vi "APDM Initialize Hardware.vi"(3 "error in (no error)":errorcluster, 4 "Gyro Sim Time Data":path=path "C:/Users/jfalesi/Desktop/CP FES Walking Code/Original/Ahad Vi/CP Code/Offline data/TD_7_time.txt", 5 "APDM Context in":T1) -> (0 "error out":errorcluster, 2 "APDM Context out":T1)   [LabVIEW 2019]
uses:
  Controls/APDM Context Cluster.ctl
  <vilib>/Utility/file.llb/Read Delimited Spreadsheet (DBL).vi
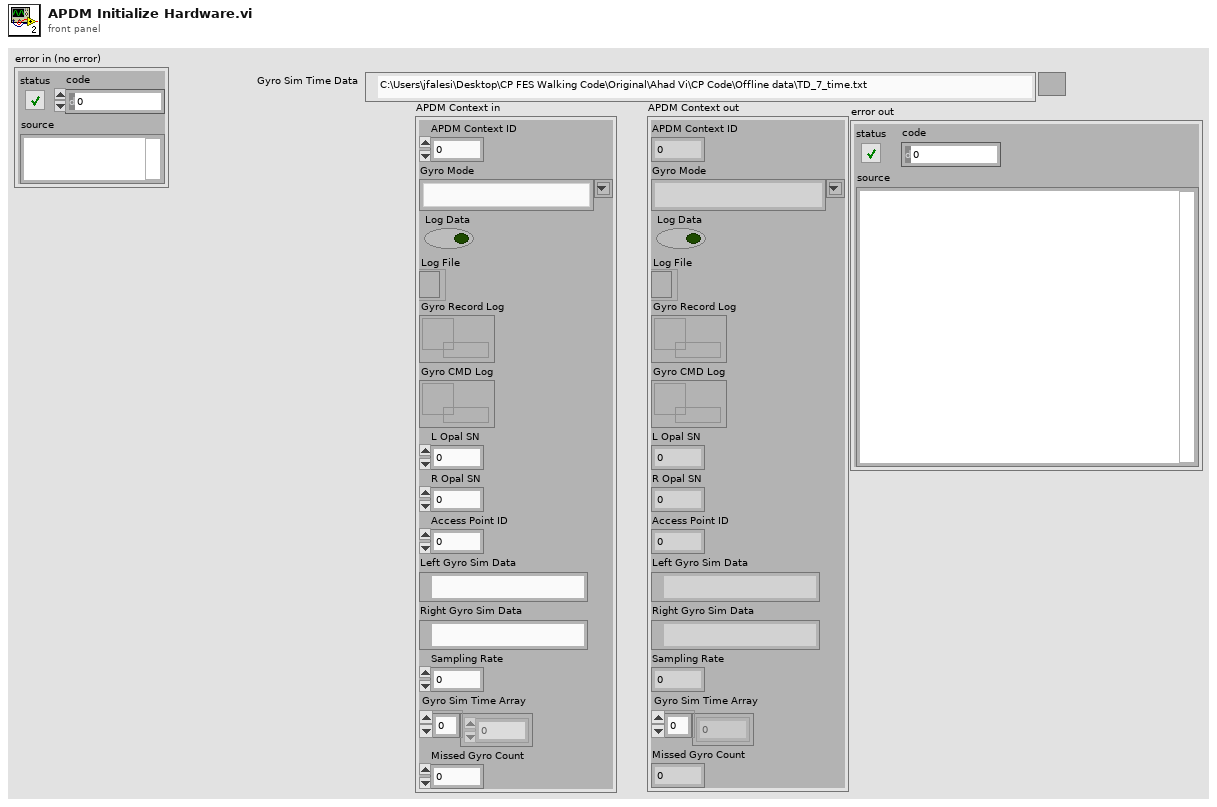
[diagram p1: front panel]
types:
  T1 = typedef "APDM Context Cluster.ctl" = cluster{"APDM Context ID":u32, "Gyro Mode":string, "Log Data":bool, "Log File":refnum<file>, "Gyro Record Log":refnum<queue>, "Gyro CMD Log":refnum<queue>, "L Opal SN":u32, "R Opal SN":u32, "Access Point ID":u32, "Left Gyro Sim Data":path, "Right Gyro Sim Data":path, "Sampling Rate":dbl, "Gyro Sim Time Array":dbl[], "Missed Gyro Count":dbl}
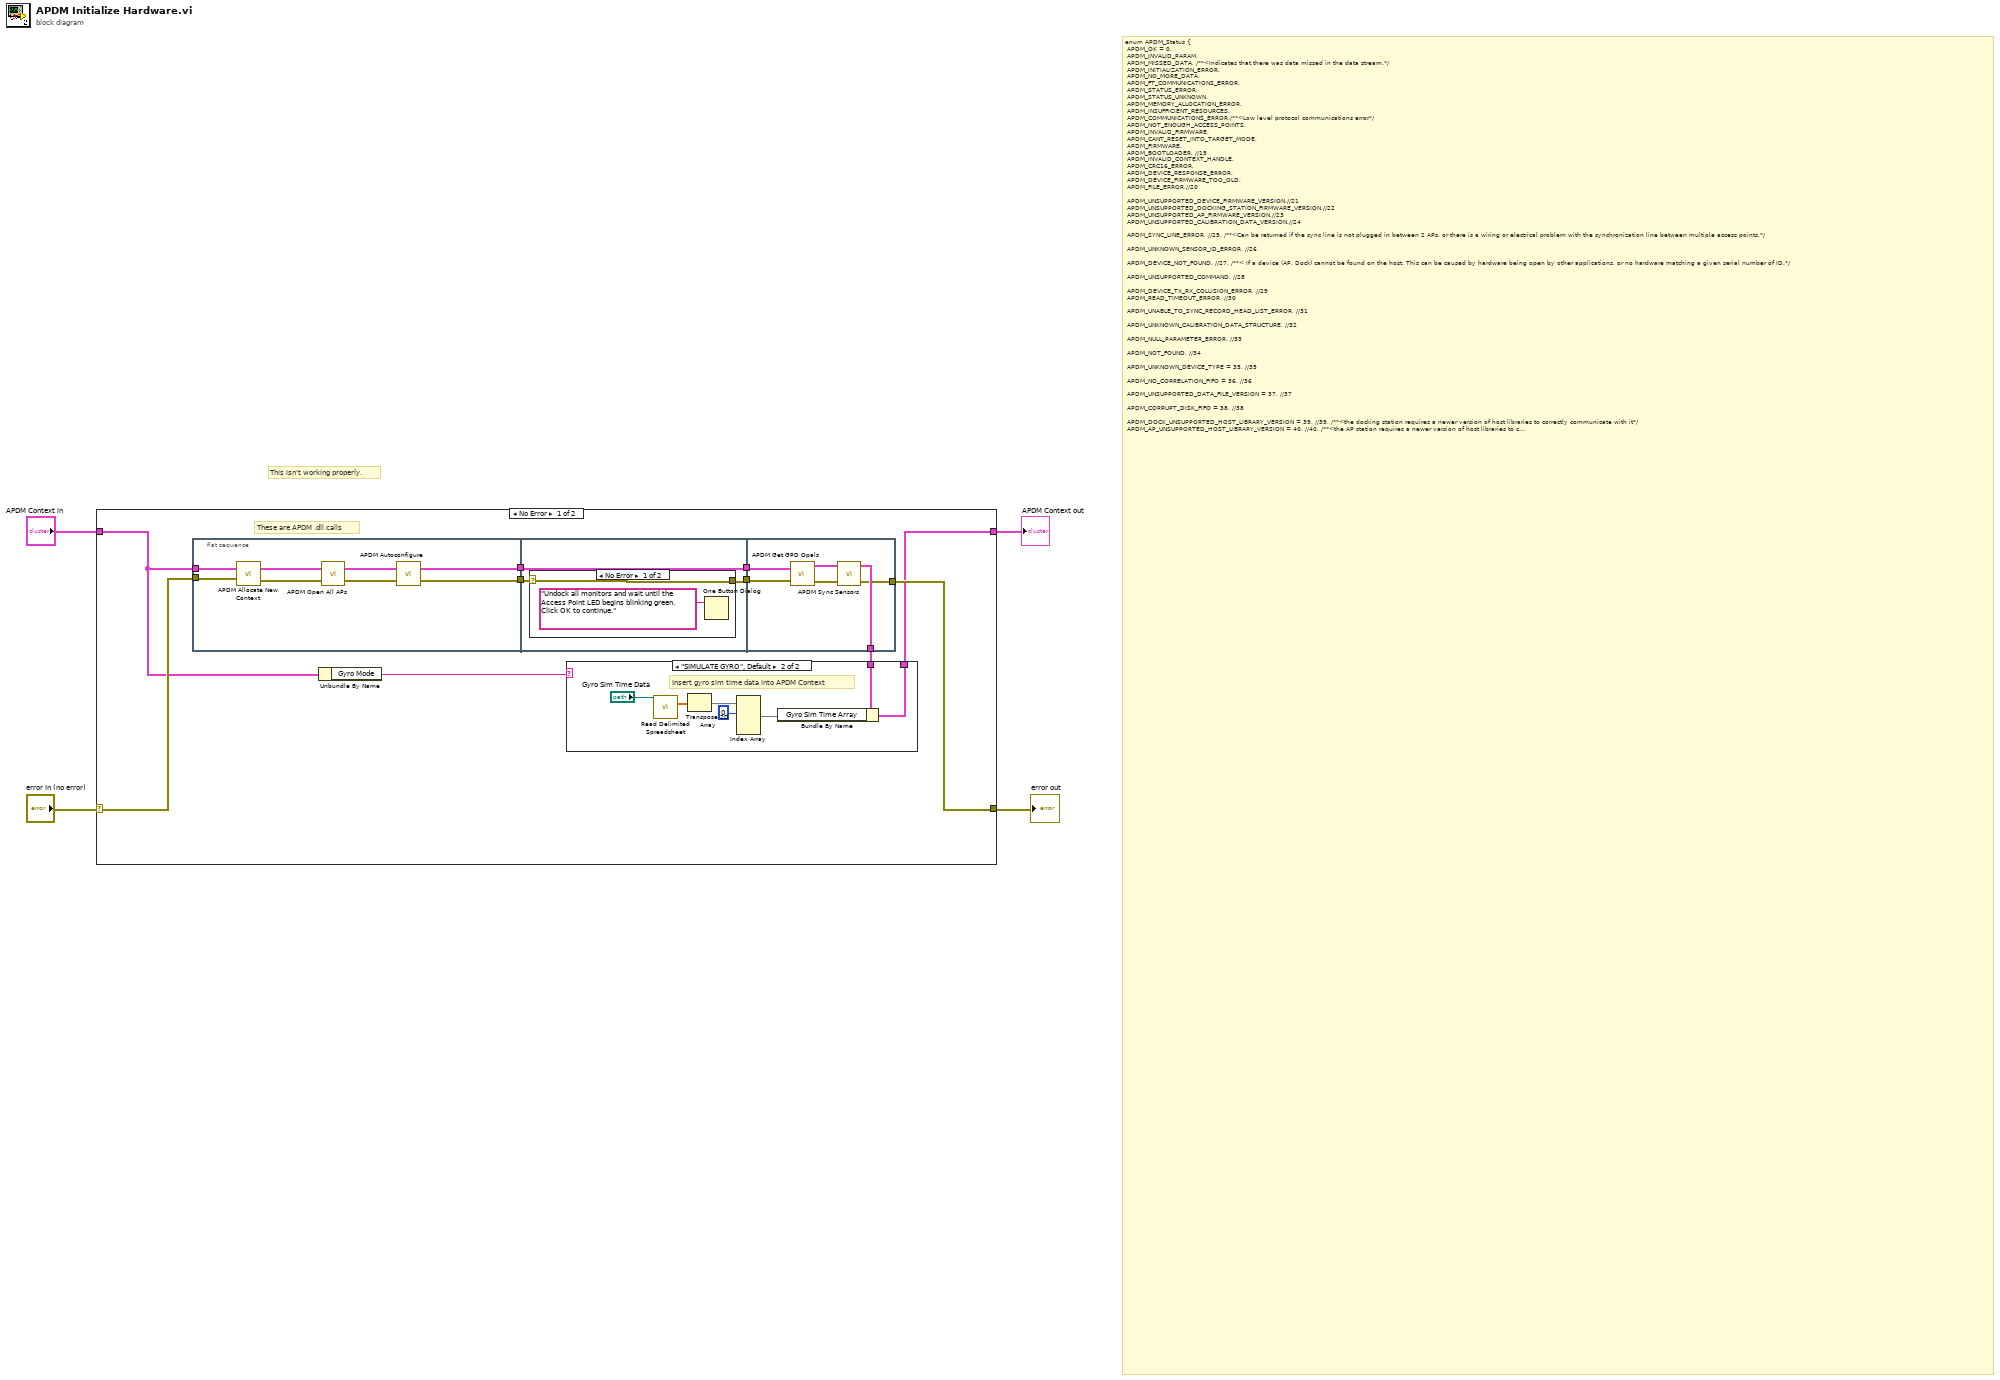
[diagram p0: block diagram]
diagram:
  # "This isn't working properly."
  # "enum APDM_Status {\n\tAPDM_OK = 0,\n\tAPDM_INVALID_PARAM,\n\tAPDM_MISSED_DATA, /**<Indicates that there was data missed in the data stream.*/\n\tAPDM_INITIALIZATION_ERROR,\n\tAPDM_NO_MORE_DATA,\n\tAPDM_FT_COMMUNICATIONS_ERROR,\n\tAPDM_STATUS_ERROR,\n\tAPDM_STATUS_UNKNOWN,\n\tAPDM_MEMORY_ALLOCATION_ERROR,\n\tAPDM_INSUFFICIENT_RESOURCES,\n\tAPDM_COMMUNICATIONS_ERROR,/**<Low level protocol communications error*/\n\tAPDM_NOT_ENOUGH_ACCESS_POINTS,\n\tAPDM_INVALID_FIRMWARE,\n\tAPDM_CANT_RESET_INTO_TARGET_MODE,\n\tAPDM_FIRMWARE,\n\tAPDM_BOOTLOADER, //15\n\tAPDM_INVALID_CONTEXT_HANDLE,\n\tAPDM_CRC16_ERROR,\n\tAPDM_DEVICE_RESPONSE_ERROR,\n\tAPDM_DEVICE_FIRMWARE_TOO_OLD,\n\tAPDM_FILE_ERROR,//20\n\n\tAPDM_UNSUPPORTED_DEVICE_FIRMWARE_VERSION,//21\n\tAPDM_UNSUPPORTED_DOCKING_STATION_FIRMWARE_VERSION,//22\n\tAPDM_UNSUPPORTED_AP_FIRMWARE_VERSION,//23\n\tAPDM_UNSUPPORTED_CALIBRATION_DATA_VERSION,//24\n\n\tAPDM_SYNC_LINE_ERROR, //25, /**<Can be returned if the sync line is not plugged in between 2 APs, or there is a wiring or electrical problem with the synchronization line between multiple access points.*/\n\n\tAPDM_UNKNOWN_SENSOR_ID_ERROR, //26\n\n\tAPDM_DEVICE_NOT_FOUND, //27, /**< If a device (AP, Dock) cannot be found on the host. This can be caused by hardware being open by other applications, or no hardware matching a given serial number of ID.*/\n\n\tAPDM_UNSUPPORTED_COMMAND, //28\n\n\tAPDM_DEVICE_TX_RX_COLLISION_ERROR, //29\n\tAPDM_READ_TIMEOUT_ERROR, //30\n\n\tAPDM_UNABLE_TO_SYNC_RECORD_HEAD_LIST_ERROR, //31\n\n\tAPDM_UNKNOWN_CALIBRATION_DATA_STRUCTURE, //32\n\n\tAPDM_NULL_PARAMETER_ERROR, //33\n\n\tAPDM_NOT_FOUND, //34\n\n\tAPDM_UNKNOWN_DEVICE_TYPE = 35, //35\n\n\tAPDM_NO_CORRELATION_FIFO = 36, //36\n\n\tAPDM_UNSUPPORTED_DATA_FILE_VERSION = 37, //37\n\n\tAPDM_CORRUPT_DISK_FIFO = 38, //38\n\n\tAPDM_DOCK_UNSUPPORTED_HOST_LIBRARY_VERSION = 39, //39, /**<the docking station requires a newer version of host libraries to correctly communicate with it*/\n\tAPDM_AP_UNSUPPORTED_HOST_LIBRARY_VERSION = 40, //40, /**<the AP station requires a newer version of host libraries to correctly communicate with it*/\n\n\tAPDM_UNEXPECTED_STRUCTURE_VALUE = 41,\n\t\n\tAPDM_BAD_DATA = 42, //42, /**< Indicates bad data detected during calibration. Either in the calibration data stored on the monitor, or in the raw data stream.*/\n\n\tAPDM_CORRUPT_CONTEXT = 43, //43 /**< If for some reason a part of the contex appears corrupt, this error code will be returned*/\n\n\tAPDM_AP_READ_TIMEOUT_ERROR = 44,\n\tAPDM_MONITOR_READ_TIMEOUT_ERROR = 45,\n\tAPDM_DOCK_READ_TIMEOUT_ERROR = 46,\n\n\n\tAPDM_DEVICE_RESPONSE_ERROR_CRC_ERROR = 47,\n\tAPDM_DEVICE_RESPONSE_ERROR_INVALID_COMMAND,\n\tAPDM_DEVICE_RESPONSE_ERROR_INVALID_PARAM_SIZE,\n\tAPDM_DEVICE_RESPONSE_ERROR_INVALID_PARAM_VALUE,\n\tAPDM_DEVICE_RESPONSE_ERROR_ERROR_EXECUTING_COMMAND,\n\n\tAPDM_RECALIBRATION_INSUFFICIENT_DATA,\n\tAPDM_RECALIBRATION_BAD_FIT,\n\tAPDM_RECALIBRATION_INSUFFICIENT_MOVEMENT,\n\n\tAPDM_FIRMWARE_COMBINATION_ERROR,\n\n\tAPDM_DATA_FROM_UNEXPECTED_MONITOR_ERROR,\n\t\n\tAPDM_ORIENTATION_ERROR,\n\n\tAPDM_UNABLE_TO_PING_MONITOR_ERROR,\n\n\tAPDM_FIRMWARE_INCOMPATABLE,\n\tAPDM_INVLAID_MONITOR_CONFIGURATION,\n\n\tAPDM_UNABLE_TO_MATCH_EXPECTED_AP_IDS,\n\n\tAPDM_AP_LIBUSB_ERROR_NO_DEVICE,\n\tAPDM_DOCK_LIBUSB_ERROR_NO_DEVICE,\n    APDM_NO_FILE_OVERLAP,\n\n\n\tAPDM_LIB_USB_ERROR = 2000,\n\tAPDM_LIBUSB_ERROR_IO = 2001,/**< Input/output error */\n\tAPDM_LIBUSB_ERROR_INVALID_PARAM = 2002,/**< Invalid parameter */\n\tAPDM_LIBUSB_ERROR_ACCESS = 2003,/**< Access denied (insufficient permissions) */\n\tAPDM_LIBUSB_ERROR_NO_DEVICE = 2004,/**< No such device (it may have been disconnected) */\n\tAPDM_LIBUSB_ERROR_NOT_FOUND = 2005,/**< Entity not found */\n\tAPDM_LIBUSB_ERROR_BUSY = 2006,/**< Resource busy */\n\tAPDM_LIBUSB_ERROR_TIMEOUT = 2007,/**< Operation timed out */\n\tAPDM_LIBUSB_ERROR_OVERFLOW = 2008,/**< Overflow */\n\tAPDM_LIBUSB_ERROR_PIPE = 2009,/**< Pipe error */\n\tAPDM_LIBUSB_ERROR_INTERRUPTED = 2010,/**< System call interrupted (perhaps due to signal) */\n\tAPDM_LIBUSB_ERROR_NO_MEM = 2011,/**< Insufficient memory */\n\tAPDM_LIBUSB_ERROR_NOT_SUPPORTED = 2012,/**< Operation not supported or unimplemented on this platform */\n\tAPDM_LIBUSB_ERROR_UNKOWN = 2098,\n\tAPDM_LIBUSB_ERROR_OTHER = 2099,/**< Other error */\n\n\tAPDM_FTDI_COMM_ERROR = 3000,\n};"
  n1 = case shown="No Error" "error in (no error)" {
    selector: "error in (no error)" -> [w7 w44]
    tunnel: [w8 w44] -> w4
    tunnel: "APDM Context in" -> [w6 w43]
    tunnel: [w5 w43] -> w1
    frame No Error {
      # "These are APDM .dll calls"
      n2 = flat-sequence {
        tunnel: w6 -> [w21]
        tunnel: [w17] -> w14
        tunnel: [w15] -> w13
        tunnel: w7 -> [w19]
        tunnel: [w25] -> w12
        tunnel: w14 -> [w25]
        tunnel: w13 -> [w24]
        tunnel: [w23] -> w11
        tunnel: w12 -> [w34]
        tunnel: [w32] -> w9
        tunnel: w11 -> [w31]
        tunnel: [w29] -> w8
        frame #0 {
          n3 = call "APDM Allocate New Context.vi"("error in (no error)"=w19, "APDM Context In"=w21) -> ("error out"=w20:errorcluster, "APDM Context Out"=w22:T1)
          n4 = call "APDM Open All APs.vi"("error in (no error)"=w20, "APDM Context"=w22) -> ("error out"=w16:errorcluster, "APDM Context"=w18:T1)
          n5 = call "APDM Autoconfigure.vi"("error in (no error)"=w16, "APDM Context"=w18) -> ("error out"=w15:errorcluster, "APDM Context"=w17:T1)
        }
        frame #1 {
          n6 = case shown="No Error" w24 {
            selector: w24 -> [w26 w28]
            tunnel: [w26 w28] -> w23
            frame No Error {
              n7 = One Button Dialog(message="Undock all monitors and wait until the Access Point LED begins blinking green. Click OK to continue.") -> ()  [unwired: 1 in, 1 out]
            }
            frame Error {
            }
          }
        }
        frame #2 {
          n8 = call "APDM Get GPD Opals.vi"("APDM Context"=w34, "error in (no error)"=w31) -> ("APDM Context"=w33:T1, "error out"=w30:errorcluster)  [unwired: 1 out]
          n9 = call "APDM Sync Sensors.vi"("error in (no error)"=w30, "APDM Context"=w33) -> ("error out"=w29:errorcluster, "APDM Context"=w32:T1)  [unwired: 2 in]
        }
      }
      n10 = Unbundle By Name(w6) -> ("Gyro Mode"=w10:string)
      n11 = case shown="\"SIMULATE GYRO\", Default" w10 {
        tunnel: [w35 w38] -> w5
        tunnel: w9 -> [w35 w36]
        frame "REAL LIVE GYRO" {
          # "REAL LIVE GYRO"
        }
        frame "SIMULATE GYRO", Default {
          # "Insert gyro sim time data into APDM Context"
          # "Stimulate"
          n12 = call-poly <vilib>:"Read Delimited Spreadsheet.vi"("file path (dialog if empty)"="Gyro Sim Time Data") -> ("all rows"=w41:dbl[][])  [unwired: 9 in, 5 out]
          n13 = Transpose 2D Array(2D array=w41) -> (transposed array=w40:dbl[][])
          n14 = Index Array(array=w40, index (row) #1=0 ("index")) -> (element #1=w37:dbl[])  [unwired: 3 in, 1 out]
          n15 = Bundle By Name(cluster=w36, "Gyro Sim Time Array"=w37) -> (w38:T1)
        }
      }
    }
    frame Error {
    }
  }
  "error out" <- w4
  "APDM Context out" <- w1
